vi "SSL_read.vi"(8 "error in (no error)":errorcluster, 10 "Bytes to read":i32, 11 "SSL in":refnum<class "SSL.lvclass">) -> (0 "error out":errorcluster, 2 "Read bytes":u8[](array[numeric]), 3 "SSL out":refnum<class "SSL.lvclass">)   [LabVIEW 2013, in "SSL_Lib.lvlib" / "SSL.lvclass"]
uses:
  SSL.lvclass
  SSL-Lib/SSL-Lib.lvclass/SSL-Lib.ctl
  SSL.lvclass/SSL.ctl
  SSL-Lib/Read SSL Library Path.vi
  Read Handle.vi
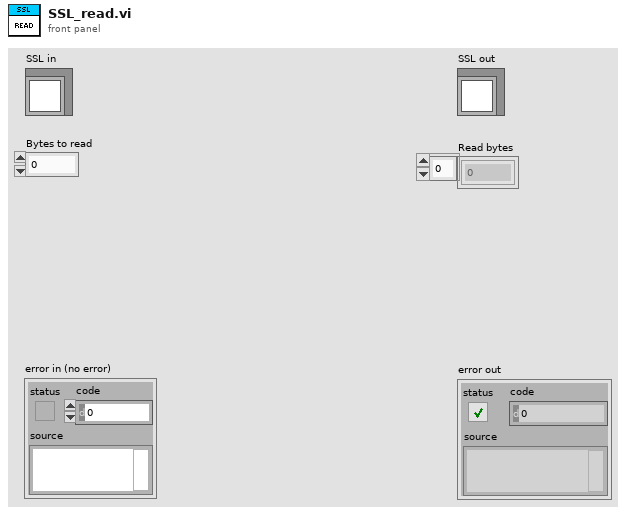
[diagram p1: front panel]
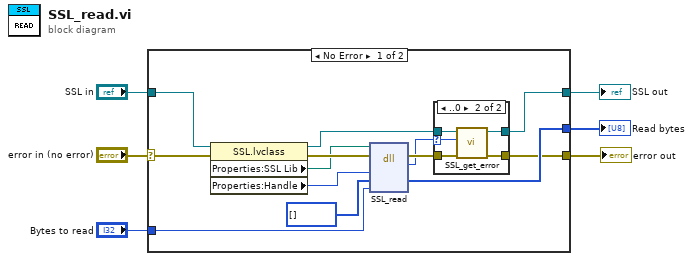
[diagram p0: block diagram]
diagram:
  n1 = case shown="No Error" "error in (no error)" {
    selector: "error in (no error)" -> [w19 w27]
    tunnel: [w8 w28] -> w4
    tunnel: "SSL in" -> [w15 w28]
    tunnel: [w10 w27] -> w3
    tunnel: [w13 _] -> w2
    tunnel: "Bytes to read" -> [w12 _]
    frame No Error {
      n2 = property class="SSL.lvclass"(reference=w15, error in=w19) -> (reference out=w9:refnum<class "SSL.lvclass">, error out=w18:errorcluster, "Properties:SSL Lib"=w17:path, "Properties:Handle"=w16:u64)
      n3 = dll-call lib="C:/Program Files (x86)/National Instruments/Shared/nissl/NIssleay32.dll" fn="SSL_read"(path in=w17, error in=w18, "SSL"=w16, "buf"=u8[] [], "num"=w12) -> (error out=w11:errorcluster, "return type"=w7:i32, "buf"=w13:u8[])  [unwired: 3 in, 1 out]
      n4 = case shown="..0" w7 {
        selector: w7 -> [_ w22]
        tunnel: w11 -> [w20 w26]
        tunnel: [w20 w25] -> w10
        tunnel: w9 -> [w21 w24]
        tunnel: [w21 w23] -> w8
        frame Default {
        }
        frame ..0 {
          n5 = call "SSL_get_error.vi"("error in (no error)"=w26, "SSL return code"=w22, "SSL-Lib in"=w24) -> ("error out"=w25:errorcluster, "SSL-Lib out"=w23:refnum<class "SSL.lvclass">)  [unwired: 6 in, 1 out]
        }
      }
    }
    frame Error {
    }
  }
  "SSL out" <- w4
  "error out" <- w3
  "Read bytes" <- w2
